vi "Get Parent Interfaces.vi"(8 "error in (no error)":errorcluster {"code" format="Error %.0f"}, 11 "Interface Documenation In":refnum<class "Interface Documenation.lvclass">) -> (0 "error out":errorcluster {"code" format="Error %.0f"}, 2 "Parent Interfaces":T1[](array[typedef]), 3 "Interface Documenation Out":refnum<class "Interface Documenation.lvclass">)   [LabVIEW 2023, in "VIDoc Parsing.lvlib" / "Interface Documenation.lvclass"]
uses:
  Interface Documenation.lvclass
  TypeDefs/Base Class Info Cluster.ctl
  <vilib>/picture/picture.llb/imagedata.ctl
  Interface Documenation.lvclass/Interface Documenation.ctl
  VIDoc Parsing.lvlib
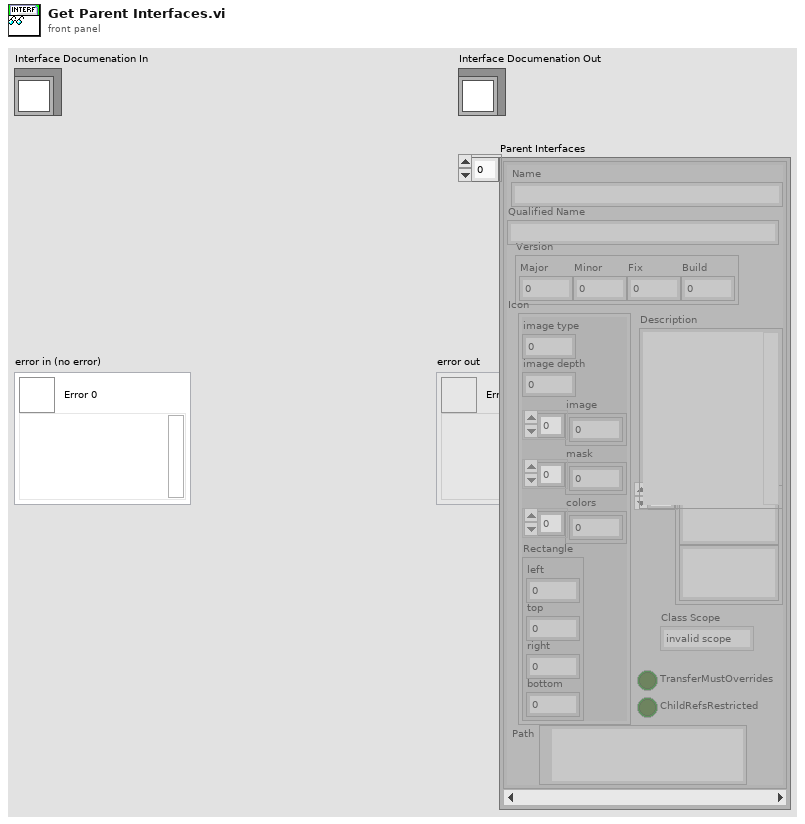
[diagram p1: front panel]
types:
  T1 = typedef "VIDoc Parsing.lvlib/Base Class Info Cluster.ctl" = cluster{"Name":string, "Icon":T2, "Version":cluster{"Major":u16, "Minor":u16, "Fix":u16, "Build":u16}, "Description":string, "Friends":string[], "ChildRefsRestricted":bool, "TransferMustOverrides":bool, "Path":path, "Qualified Name":string, "Class Scope":enum32{"invalid scope", "public", "private", "protected", "community"}}
  T2 = typedef "imagedata.ctl" = cluster{"image type":i32, "image depth":i32, "image":u8[], "mask":u8[], "colors":u32[], "Rectangle":cluster{"left":i16, "top":i16, "right":i16, "bottom":i16}}
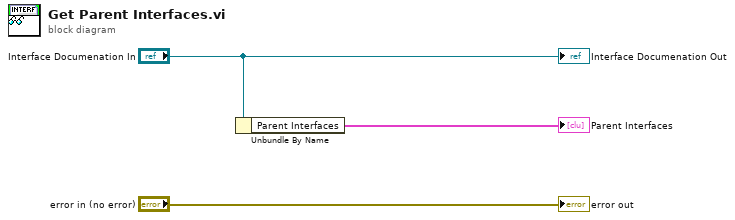
[diagram p0: block diagram]
diagram:
  n1 = Unbundle By Name("Interface Documenation In") -> ("Parent Interfaces"=→"Parent Interfaces":T1[])
  "error out" <- "error in (no error)"
  "Interface Documenation Out" <- "Interface Documenation In"
